vi "TargetSetup[Pxi linux].vi"() -> ()   [LabVIEW 2020]
uses:
  <vilib>/nisyscfg/Software 1.2.ctl
  <vilib>/nisyscfg/Component Type.ctl
  <vilib>/nisyscfg/Format With Base System Image.vi
  <vilib>/nisyscfg/Close (System).vi
  <vilib>/nisyscfg/nisyscfg.lvlib
panel:
  out "error out":errorcluster
  in  "error in (no error)":errorcluster
  in  "Target (localhost)":refnum<k21>="localhost"
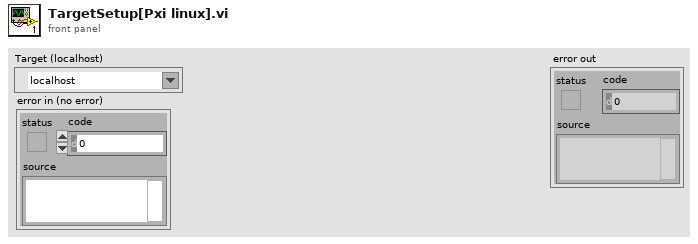
[diagram p1: front panel]
types:
  T1 = typedef "nisyscfg.lvlib/Software 1.2.ctl" = cluster{"title":string, "description":string, "ID":string, "version":string, "component type":T2}
  T2 = typedef "nisyscfg.lvlib/Component Type.ctl" = u32
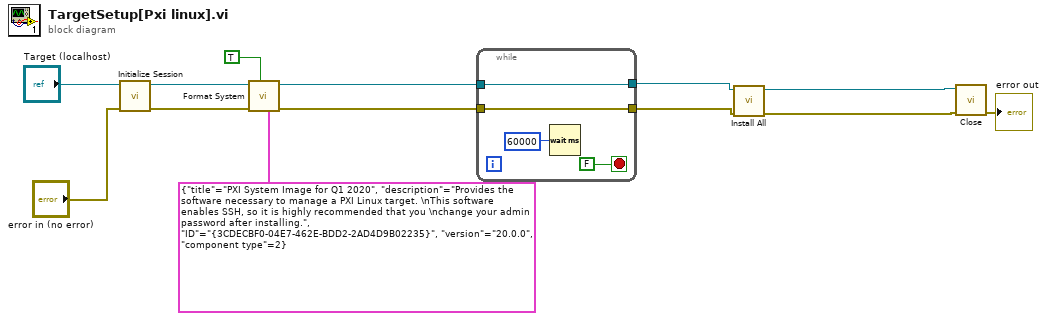
[diagram p0: block diagram]
diagram:
  n1 = call <vilib>:"Initialize Session.vi"("error in (no error)"="error in (no error)", "Target (localhost)"="Target (localhost)") -> ("error out"=w11:errorcluster, "Session out"=w10:refnum<k21>)  [unwired: 8 in]
  n2 = call-poly <vilib>:"Format System.vi"("Base System Image"=T1 {"title"="PXI System Image for Q1 2020", "description"="Provides the software necessary to manage a PXI Linux target. \nThis software enables SSH, so it is highly recommended that you \nchange your admin password after installing.", "ID"="{3CDECBF0-04E7-462E-BDD2-2AD4D9B02235}", "version"="20.0.0", "component type"=2}, "Restart Automatically (T)"=TRUE, "error in (no error)"=w11, "Session in"=w10) -> ("error out"=w5:errorcluster, "Session out"=w7:refnum<k21>)  [unwired: 6 in]
  n3 = while {
    tunnel: w7 -> [w17]
    tunnel: [w17] -> w6
    tunnel: w5 -> [w16]
    tunnel: [w16] -> w4
    stop <- FALSE stop-if-true
    n4 = Wait (ms)(milliseconds to wait=u32 60000) -> ()  [unwired: 1 out]
  }
  n5 = call <vilib>:"Install All.vi"("error in (no error)"=w4, "Session in"=w6) -> ("error out"=w2:errorcluster, "Session out"=w3:refnum<k21>)  [unwired: 6 in, 2 out]
  n6 = call-poly <vilib>:"Close.vi"("error in (no error)"=w2, "Session in"=w3) -> ("error out"=→"error out":errorcluster)  [unwired: 9 in]
